vi "Initialize XNET Tree.vi"(8 "error in":errorcluster, 9 "XNET Cluster":refnum<k21>, 10 "XNET Database":refnum<k21>, 11 "Tree":refnum<vi>) -> (0 "error out":errorcluster, 1 "Parent":string, 2 "XNET Cluster Out":refnum<k21>, 3 "Tree Out":refnum<vi>)   [LabVIEW 2013, in "J1939 Addon System Explorer.lvlib"]
uses:
  J1939 Addon System Explorer.lvlib
  <resource>/objmgr/xnet.rc
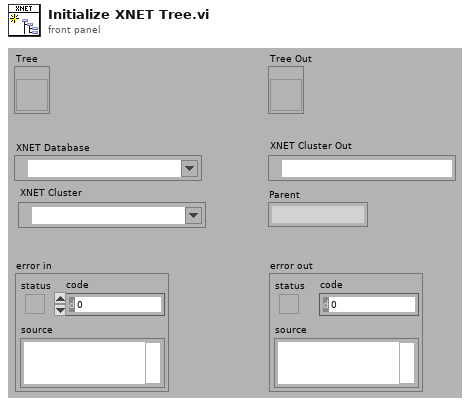
[diagram p1: front panel]
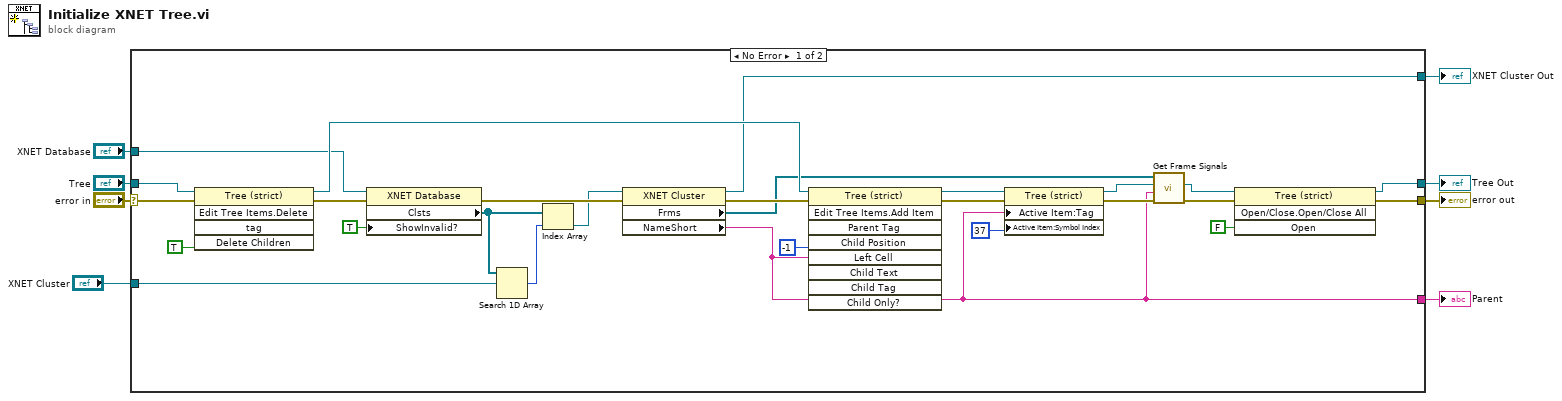
[diagram p0: block diagram]
diagram:
  n1 = case shown="No Error" "error in" {
    selector: "error in" -> [w24 w38]
    tunnel: "Tree" -> [w34 w37]
    tunnel: [w21 w38] -> w7
    tunnel: "XNET Database" -> [w17 _]
    tunnel: [w20 w37] -> w4
    tunnel: [w23 w36] -> w3
    tunnel: "XNET Cluster" -> [w13 w36]
    tunnel: [w9 _] -> w1
    frame No Error {
      n2 = invoke on="Invoke Node" class="Tree (strict)" method="Edit Tree Items.Delete"(reference=w34, error in=w24, "Delete Children"=TRUE ("Delete Children?")) -> (reference out=w35:refnum<vi>, error out=w15:errorcluster)  [unwired: 2 in, 3 out]
      n3 = property class="XNET Database"(reference=w17, error in=w15, "ShowInvalid?"=TRUE ("Show Invalid From Open?")) -> (error out=w14:errorcluster, "Clsts"=w11:refnum<k21>[])  [unwired: 1 out]
      n4 = Search 1D Array(1D array=w11, element=w13) -> (index of element=w12:i32)  [unwired: 1 in]
      n5 = Index Array(array=w11, index=w12) -> (element=w10:refnum<k21>)
      n6 = property class="XNET Cluster"(reference=w10, error in=w14) -> (reference out=w23:refnum<k21>, error out=w26:errorcluster, "Frms"=w25:refnum<k21>[], "NameShort"=w9:string)
      n7 = invoke on="Invoke Node" class="Tree (strict)" method="Edit Tree Items.Add Item"(reference=w35, error in=w26, "Child Position"=-1, "Left Cell"=w9, "Child Tag"=w9) -> (reference out=w29:refnum<vi>, error out=w28:errorcluster)  [unwired: 4 in, 7 out]
      n8 = property class="Tree (strict)"(reference=w29, error in=w28, "Active Item:Tag"=w9, "Active Item:Symbol Index"=37) -> (reference out=w30:refnum<vi>, error out=w31:errorcluster)
      n9 = call "Get Frame Signals.vi"("error in"=w31, "Parent Tag"=w9, "Tree Reference"=w30, "Frms"=w25) -> ("error out"=w19:errorcluster, "Tree Reference Out"=w18:refnum<vi>)  [unwired: 6 in]
      n10 = invoke on="Invoke Node" class="Tree (strict)" method="Open/Close.Open/Close All"(reference=w18, error in=w19, "Open"=FALSE ("Open?")) -> (reference out=w20:refnum<vi>, error out=w21:errorcluster)  [unwired: 1 in, 2 out]
    }
    frame Error {
    }
  }
  "error out" <- w7
  "Tree Out" <- w4
  "XNET Cluster Out" <- w3
  "Parent" <- w1
